vi "Calc Data.vi"(0 "DATA in":T1, 7 "Value":dbl) -> (4 "DATA iout":T1)   [LabVIEW 2019, in "OscillationDetector.lvclass"]
uses:
  OscillationDetector.lvclass
  DATA Oscill.ctl
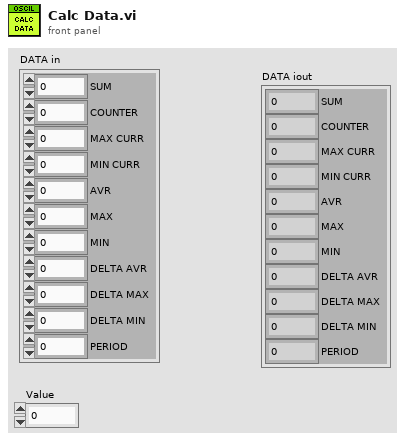
[diagram p1: front panel]
types:
  T1 = typedef "DATA Oscill.ctl" = cluster{"SUM":dbl, "COUNTER":dbl, "MAX CURR":dbl, "MIN CURR":dbl, "AVR":dbl, "MAX":dbl, "MIN":dbl, "DELTA AVR":dbl, "DELTA MAX":dbl, "DELTA MIN":dbl, "PERIOD":dbl}
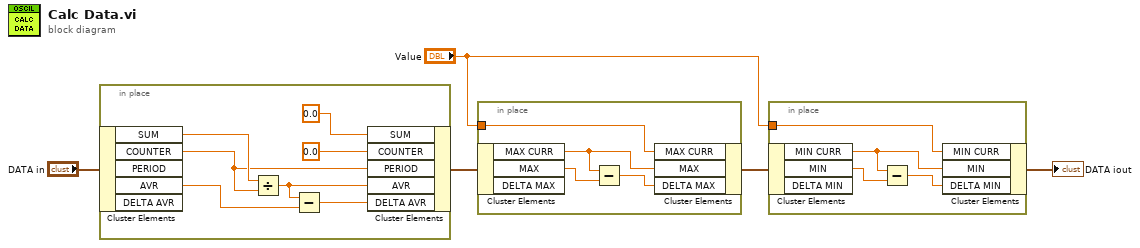
[diagram p0: block diagram]
diagram:
  n1 = in-place {
    n2 = in-place-cluster #1("DATA in") -> ("SUM"=w12:dbl, "COUNTER"=w6:dbl, "AVR"=w11:dbl)  [unwired: 2 out]
    n3 = Divide(x=w12, y=w6) -> (x/y=w8:dbl)
    n4 = Subtract(x=w8, y=w11) -> (x-y=w7:dbl)
    n5 = in-place-cluster #1("SUM"=0.0, "COUNTER"=0.0, "PERIOD"=w6, "AVR"=w8, "DELTA AVR"=w7) -> (w4:T1)
  }
  n6 = in-place {
    in-place-border: "Value" -> [w13]
    n7 = in-place-cluster #2(w4) -> ("MAX CURR"=w15:dbl, "MAX"=w14:dbl)  [unwired: 1 out]
    n8 = Subtract(x=w15, y=w14) -> (x-y=w16:dbl)
    n9 = in-place-cluster #2("MAX CURR"=w13, "MAX"=w15, "DELTA MAX"=w16) -> (w3:T1)
  }
  n10 = in-place {
    in-place-border: "Value" -> [w17]
    n11 = in-place-cluster #3(w3) -> ("MIN CURR"=w19:dbl, "MIN"=w18:dbl)  [unwired: 1 out]
    n12 = Subtract(x=w19, y=w18) -> (x-y=w20:dbl)
    n13 = in-place-cluster #3("MIN CURR"=w17, "MIN"=w19, "DELTA MIN"=w20) -> (→"DATA iout":T1)
  }
